vi "Boiler Controller.vi"(8 "Error In":errorcluster, 11 "Message Queues":T1) -> (0 "Error Out":errorcluster)   [LabVIEW 2015]
uses:
  support/Message Queue/All Message Queues.ctl
  support/Message Queue/Message Cluster.ctl
  support/Message Queue/Message Queue.lvlib
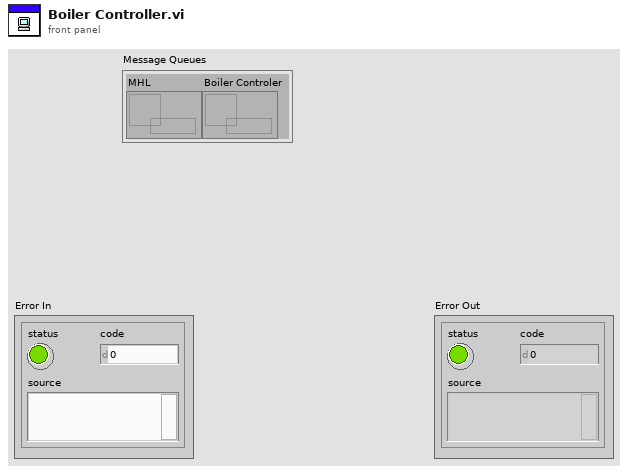
[diagram p1: front panel]
types:
  T1 = typedef "Message Queue.lvlib/All Message Queues.ctl" = cluster{"MHL":refnum<queue>, "Boiler Controler":refnum<queue>}
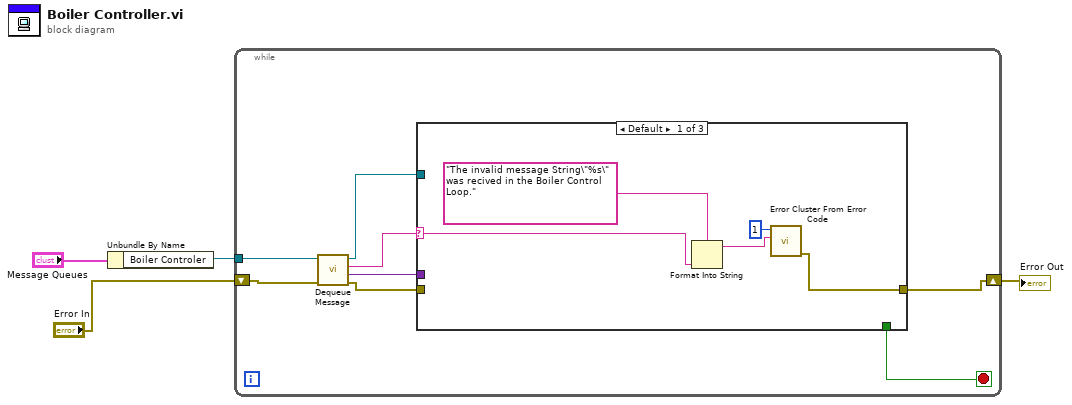
[diagram p0: block diagram]
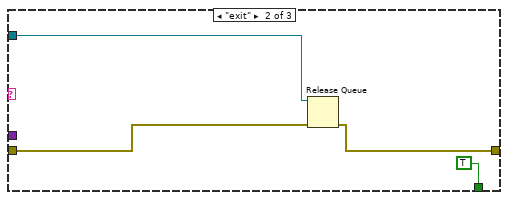
[diagram p2: hidden frame]
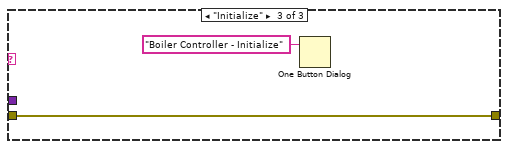
[diagram p3: hidden frame]
diagram:
  n1 = Unbundle By Name("Message Queues") -> ("Boiler Controler"=w3:refnum<queue>)
  n2 = while {
    tunnel: w3 -> [w12]
    shift-right: [w7] -> w1
    shift-left: "Error In" -> [w11]
    stop <- w5 stop-if-true
    n3 = call "Dequeue Message.vi"("error in (no error)"=w11, "Message Queue"=w12) -> ("error out"=w6:errorcluster, "Message Data"=w8:variant, "Message"=w9:string, "dup Message Queue"=w10:refnum<queue>)  [unwired: 6 in]
    n4 = case shown="Default" w9 {
      selector: w9 -> [w13 _ _]
      tunnel: w10 -> [_ w19 _]
      tunnel: w8 -> [_ _ _]
      tunnel: [w15 w20 w22] -> w7
      tunnel: w6 -> [_ w21 w22]
      tunnel: [_ TRUE _] -> w5
      frame Default {
        n5 = Format Into String(format string="The invalid message String\"%s\" was recived in the Boiler Control Loop.", w13) -> (resulting string=w14:string)  [unwired: 2 in, 1 out]
        n6 = call <vilib>:"Error Cluster From Error Code.vi"("error message (\"\")"=w14, "error code (0)"=1) -> ("error out"=w15:errorcluster)  [unwired: 7 in]
      }
      frame "exit" {
        n7 = Release Queue(queue=w19, error in (no error)=w21) -> (error out=w20:errorcluster)  [unwired: 1 in, 2 out]
      }
      frame "Initialize" {
        n8 = One Button Dialog(message="Boiler Controller - Initialize") -> ()  [unwired: 1 in, 1 out]
      }
    }
  }
  "Error Out" <- w1
